vi "Track_Node.vi"   [LabVIEW 2020]
uses:
  <vilib>/Rock Robotics/Network Tables/NT Write Number.vi
  Robot Global Data.vi
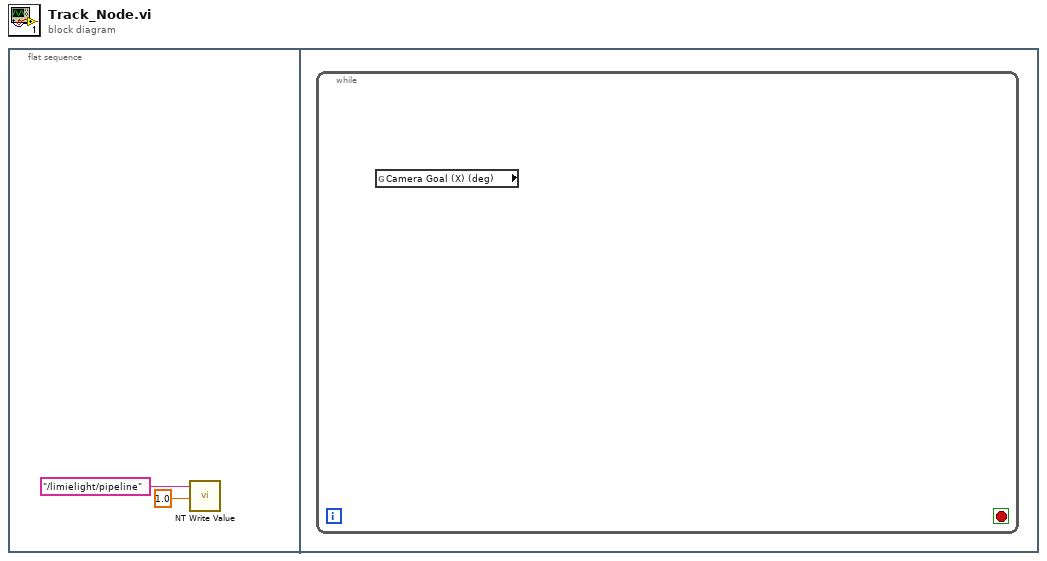
[diagram p0: block diagram]
diagram:
  n1 = flat-sequence {
    frame #0 {
      n2 = call-poly <vilib>:"NT Write Value.vi"("value"=1.0, "name"="/limielight/pipeline") -> ()  [unwired: 9 in, 1 out]
    }
    frame #1 {
      n3 = while {
        stop <- _ stop-if-true
        n4 = global read "Robot Global Data.vi" "Camera Goal (X) (deg)"() -> ()  [unwired: 1 out]
      }
    }
  }
